vi "Pause.vi"(8 "error in (no error)":errorcluster, 11 "Ismatech Settings In":T1={"VISA resource name"="", "Simulated?"=FALSE, "Pump Number"=1.0, "Reverse?"=FALSE} {"Pump Number" min=1.0 max=20.0 step=1.0}) -> (0 "error out":errorcluster, 1 "Connection Error":bool, 3 "Ismatech Settings Out":T1={"VISA resource name"="", "Simulated?"=FALSE, "Pump Number"=1.0, "Reverse?"=FALSE} {"Pump Number" min=1.0 max=20.0 step=1.0})   [LabVIEW 2018, in "Ismatec ISM 831C.lvlib"]
uses:
  Ismatec ISM 831C.lvlib
  Controls/Ismatech ISM831C Settings Cluster.ctl
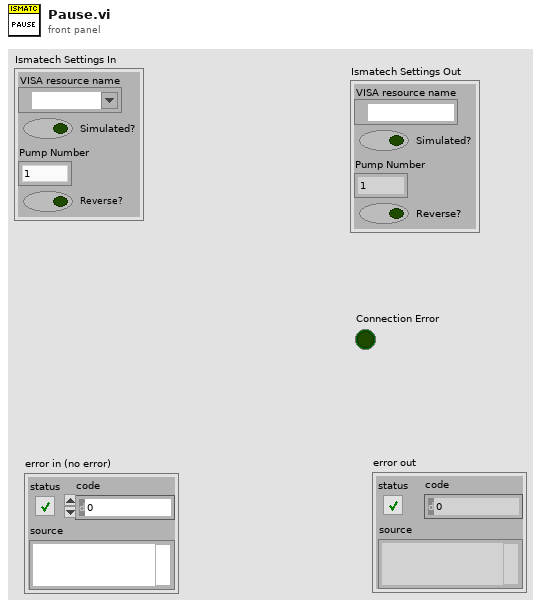
[diagram p1: front panel]
types:
  T1 = typedef "Ismatec ISM 831C.lvlib/Ismatech ISM831C Settings Cluster.ctl" = cluster{"VISA resource name":refnum<visa-resource-name>, "Simulated?":bool, "Pump Number":dbl, "Reverse?":bool}
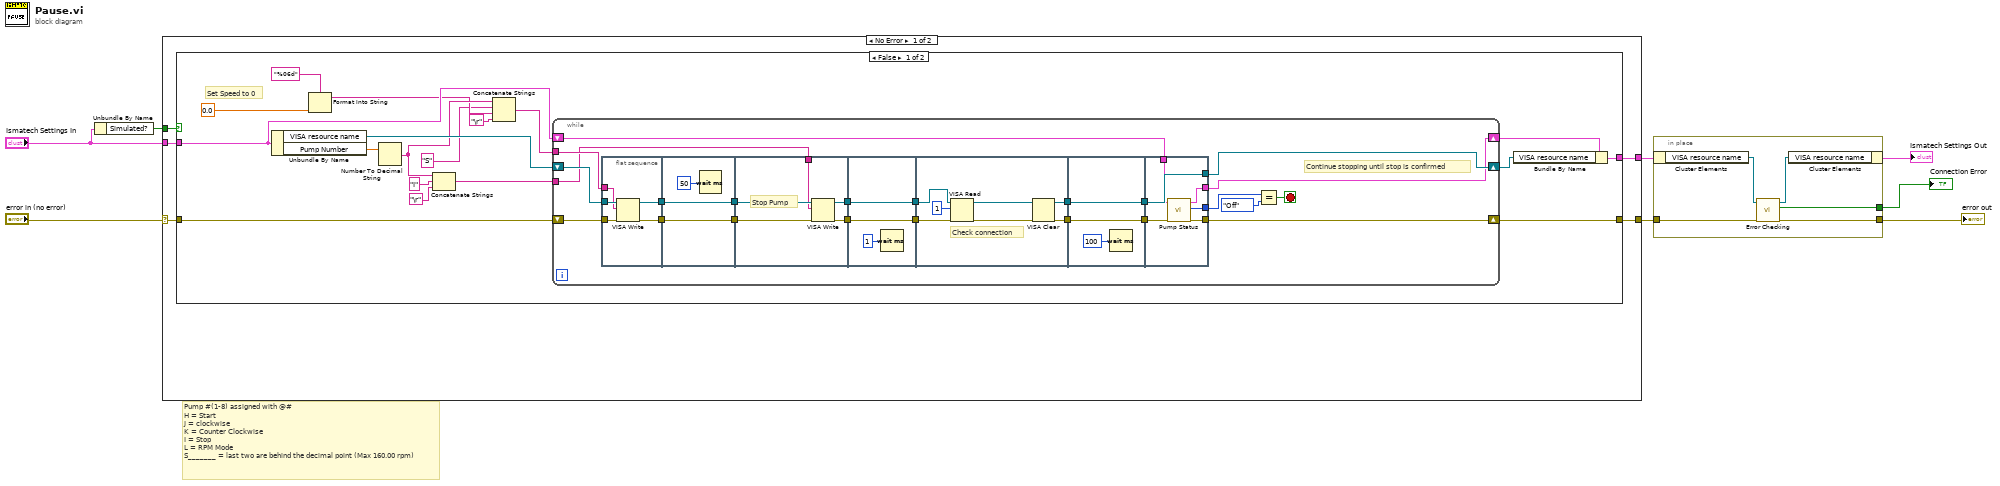
[diagram p0: block diagram]
diagram:
  # "Pump #(1-8) assigned with @#\nH = Start\nJ = clockwise\nK = Counter Clockwise\nI = Stop\nL = RPM Mode\nS_______ = last two are behind the decimal point (Max 160.00 rpm)"
  n1 = Unbundle By Name("Ismatech Settings In") -> ("Simulated?"=w6:bool)
  n2 = case shown="No Error" "error in (no error)" {
    selector: "error in (no error)" -> [w11 w90]
    tunnel: [w10 w89] -> w3
    tunnel: [w9 w90] -> w5
    tunnel: "Ismatech Settings In" -> [w13 w89]
    tunnel: w6 -> [w12 _]
    frame No Error {
      n3 = case shown="False" w12 {
        tunnel: w13 -> [w24 w88]
        tunnel: [w31 w88] -> w10
        tunnel: w11 -> [w28 w87]
        tunnel: [w30 w87] -> w9
        frame False {
          # "Set Speed to 0"
          n4 = Unbundle By Name(w24) -> ("VISA resource name"=w27:refnum<visa-resource-name>, "Pump Number"=w26:dbl)
          n5 = Format Into String(format string="%06d", 0.0 ("x")) -> (resulting string=w22:string)  [unwired: 2 in, 1 out]
          n6 = Number To Decimal String(number=w26) -> (decimal integer string=w25:string)  [unwired: 1 in]
          n7 = Concatenate Strings(w25, "I", "\r") -> (w14:string)
          n8 = Concatenate Strings(w25, "S" ("string"), w22, "\r") -> (w17:string)
          n9 = while {
            shift-right: [w42] -> w30
            shift-left: w28 -> [w40]
            shift-right: [w41] -> w29
            shift-left: w27 -> [w39]
            shift-right: [w37] -> w23
            shift-left: w24 -> [w38]
            tunnel: w17 -> [w33]
            tunnel: w14 -> [w32]
            stop <- w36 stop-if-true
            # "Continue stopping until stop is confirmed"
            n10 = flat-sequence {
              tunnel: [w59] -> w54
              tunnel: [w58] -> w53
              tunnel: w40 -> [w57]
              tunnel: w39 -> [w56]
              tunnel: w33 -> [w55]
              tunnel: [w62] -> w52
              tunnel: w54 -> [w62]
              tunnel: w53 -> [w61]
              tunnel: [w61] -> w51
              tunnel: w52 -> [w65]
              tunnel: w51 -> [w64]
              tunnel: [w67] -> w50
              tunnel: [w66] -> w49
              tunnel: w32 -> [w63]
              tunnel: w50 -> [w70]
              tunnel: w49 -> [w69]
              tunnel: [w70] -> w48
              tunnel: [w69] -> w47
              tunnel: w48 -> [w77]
              tunnel: w47 -> [w75]
              tunnel: [w71] -> w46
              tunnel: [w73] -> w45
              tunnel: w46 -> [w80]
              tunnel: w45 -> [w79]
              tunnel: [w80] -> w44
              tunnel: [w79] -> w43
              tunnel: [w86] -> w41
              tunnel: [w82] -> w42
              tunnel: w44 -> [w83]
              tunnel: w43 -> [w86]
              tunnel: w38 -> [w85]
              tunnel: [w84] -> w37
              tunnel: [w81] -> w35
              frame #0 {
                n11 = VISA Write(VISA resource name=w56, write buffer=w55, error in (no error)=w57) -> (VISA resource name out=w59:refnum<visa-resource-name>, error out=w58:errorcluster)  [unwired: 1 out]
              }
              frame #1 {
                n12 = Wait (ms)(milliseconds to wait=u32 50) -> ()  [unwired: 1 out]
              }
              frame #2 {
                # "Stop Pump"
                n13 = VISA Write(VISA resource name=w65, write buffer=w63, error in (no error)=w64) -> (VISA resource name out=w66:refnum<visa-resource-name>, error out=w67:errorcluster)  [unwired: 1 out]
              }
              frame #3 {
                n14 = Wait (ms)(milliseconds to wait=u32 1) -> ()  [unwired: 1 out]
              }
              frame #4 {
                # "Check connection"
                n15 = VISA Read(VISA resource name=w75, byte count=u32 1, error in (no error)=w77) -> (VISA resource name out=w74:refnum<visa-resource-name>, error out=w72:errorcluster)  [unwired: 2 out]
                n16 = VISA Clear(VISA resource name=w74, error in (no error)=w72) -> (VISA resource name out=w73:refnum<visa-resource-name>, error out=w71:errorcluster)
              }
              frame #5 {
                n17 = Wait (ms)(milliseconds to wait=u32 100) -> ()  [unwired: 1 out]
              }
              frame #6 {
                n18 = call "Pump Status.vi"("error in (no error)"=w83, "Ismatech Settings In"=w85) -> ("error out"=w82:errorcluster, "Pump On?"=w81:enum16{"Off", "On", "Not Initialized"}, "Ismatech Settings Out"=w84:T1)  [unwired: 6 in, 1 out]
              }
            }
            n19 = Equal?(x=w35, y=enum16{"Off", "On", "Not Initialized"}."Off") -> (x = y?=w36:bool)
          }
          n20 = Bundle By Name(cluster=w23, "VISA resource name"=w29) -> (w31:T1)
        }
        frame True {
        }
      }
    }
    frame Error {
    }
  }
  n21 = in-place {
    in-place-border: w5 -> [w95]
    in-place-border: [w94] -> w4
    in-place-border: [w91] -> w1
    n22 = in-place-cluster #1(w3) -> ("VISA resource name"=w93:refnum<visa-resource-name>)
    n23 = call "Error Checking.vi"("error in (no error)"=w95, "VISA resource name"=w93) -> ("error out"=w91:errorcluster, "Connection Error"=w94:bool, "VISA resource name"=w92:refnum<visa-resource-name>)  [unwired: 7 in]
    n24 = in-place-cluster #1("VISA resource name"=w92) -> (→"Ismatech Settings Out":T1)
  }
  "Connection Error" <- w4
  "error out" <- w1
